vi "Auto Shoot.vi"(8 "Hood?":dbl, 9 "Trigger Power":dbl, 10 "RPM":dbl) -> ()   [LabVIEW 2016]
uses:
  Robot Global Data.vi
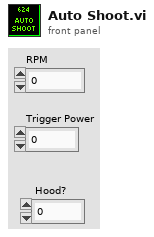
[diagram p1: front panel]
types:
  T1 = typedef "Shooter Control Cluster'.ctl" = cluster{"Shooter Modes":T2, "Shooter Commands":T3, "Manual Control Cluster":T4, "Shot Type":T5, "Agitator Power":dbl}
  T2 = typedef "Shooter Modes.ctl" = enum16{"Auto", "Manual"}
  T3 = typedef "Shooter Commands.ctl" = enum16{"Idle ", "Warmup ", "Shoot"}
  T4 = typedef "Manual Shoot Cluster.ctl" = cluster{"Shooter Power":dbl, "Hood Down?":bool, "Trigger Power":dbl}
  T5 = typedef "Shot Type.ctl" = enum16{"Vision Shot", "Dist Shot", "Key Shot"}
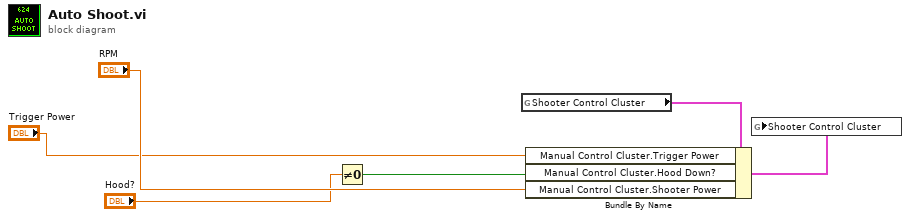
[diagram p0: block diagram]
diagram:
  n1 = Not Equal To 0?(x="Hood?") -> (x != 0?=w2:bool)
  n2 = global read "Robot Global Data.vi" "Shooter Control Cluster"() -> (w6:T1)
  n3 = Bundle By Name(cluster=w6, "Manual Control Cluster.Trigger Power"="Trigger Power", "Manual Control Cluster.Hood Down?"=w2, "Manual Control Cluster.Shooter Power"="RPM") -> (w5:T1)
  n4 = global write "Robot Global Data.vi" "Shooter Control Cluster"(w5) -> ()
